vi "main.vi"() -> ()   [LabVIEW 2015]
panel:
  out "Lines Cleared":dbl
  out "score":dbl
  out "rotation":dbl
  in  "Stop":bool
  out "Stop Variable":bool
  out "X Direction":i32
  out "Y Direction":i32
  out "Array":bool[][](array[boolean])
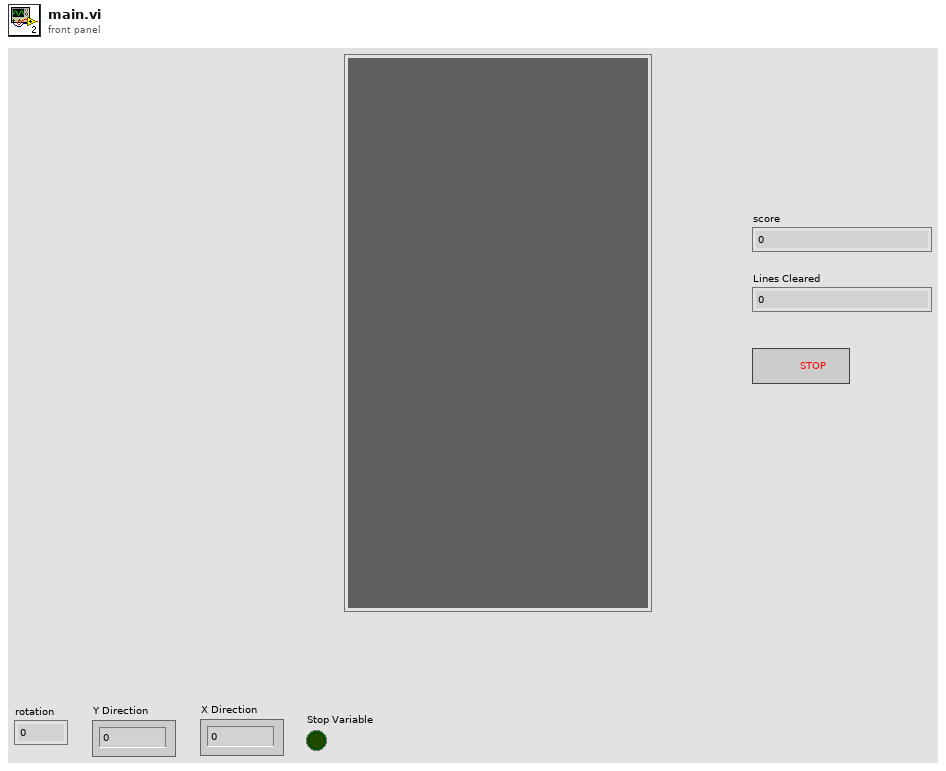
[diagram p1: front panel]
types:
  T1 = typedef "eventvkey.ctl" = enum16{"ASCII", "Enter", "Return", "Shift", "Ctrl", "Alt", "Cmd", "Opt", "Caps", "NumLock", "Clear", "Break", "Up", "Down", "Left", "Right", "Insert", "Delete", "Home", "End", "PageUp", "PageDown", "Escape", "Help", "Pause", "ScrollLock", "F1", "F2", "F3", "F4", "F5", "F6", "F7", "F8", "F9", "F10", "F11", "F12", "F13", "F14", "F15", "F16", "F17", "F18", "F19", "F20", "F21", "F22", "F23", "F24", "Play", "VolumeUp", "VolumeDown", "Mute", "Two Byte Char"}
  T2 = typedef "block.ctl" = cluster{"points":dbl[][], "type":u16, "orientaion":u16}
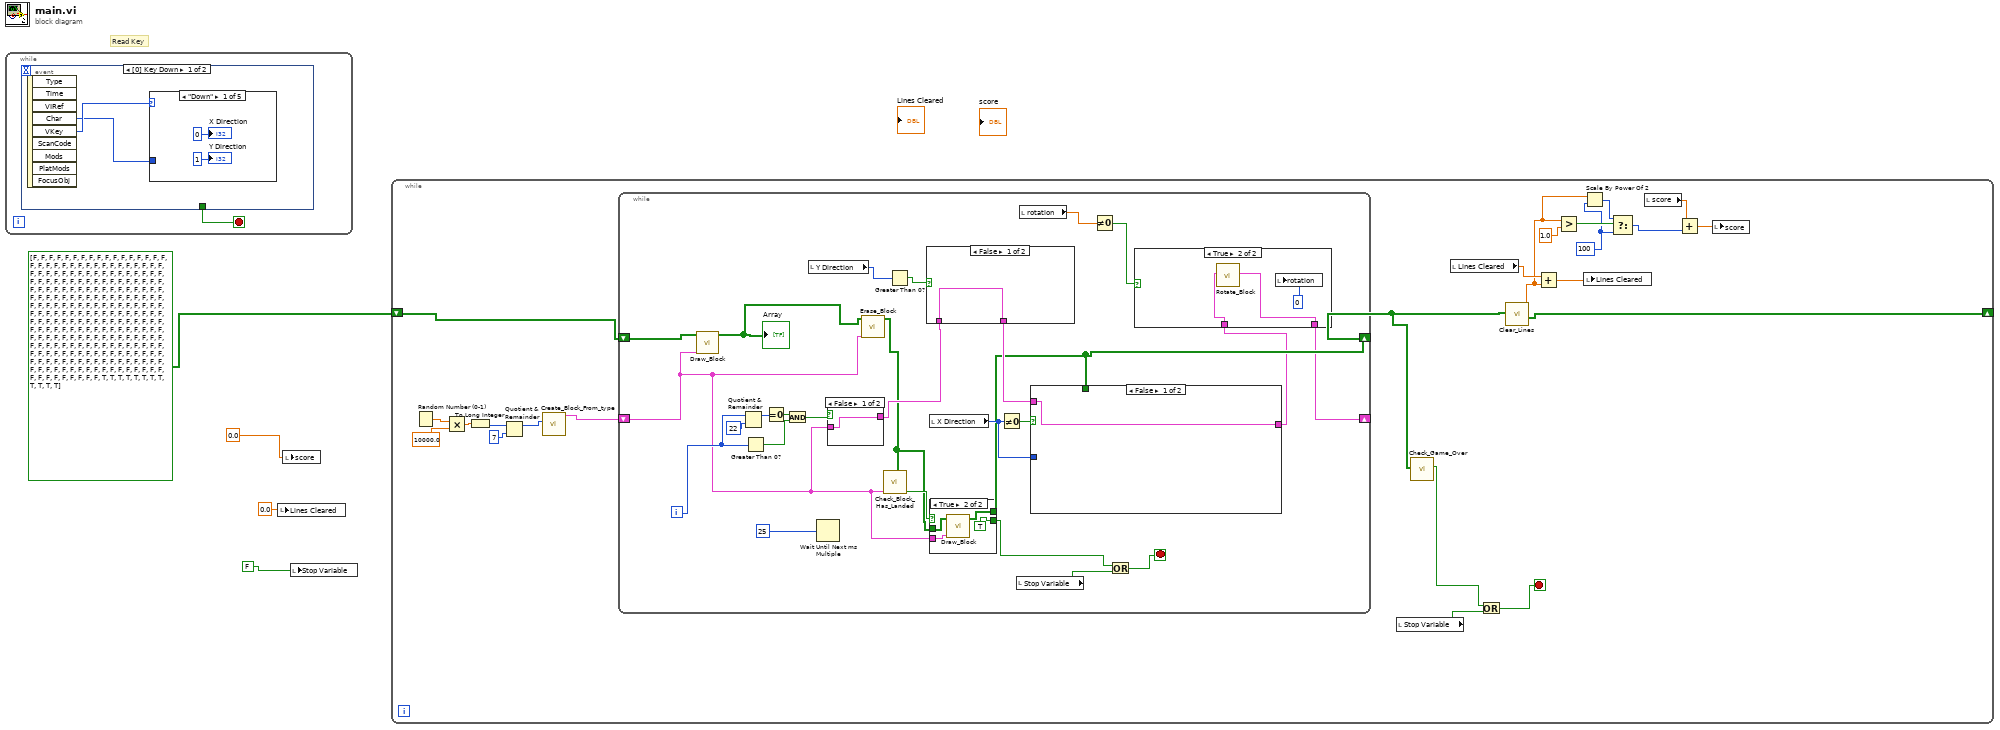
[diagram p0: block diagram]
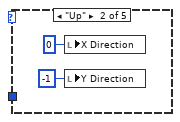
[diagram p2: hidden frame]
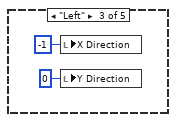
[diagram p3: hidden frame]
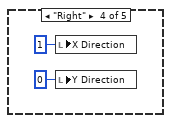
[diagram p4: hidden frame]
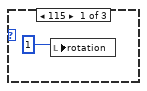
[diagram p6: hidden frame]
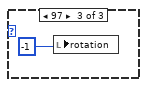
[diagram p7: hidden frame]
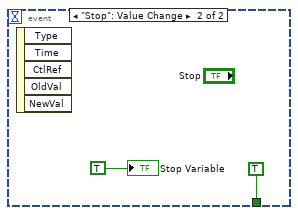
[diagram p8: hidden frame]
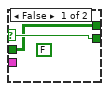
[diagram p10: hidden frame]
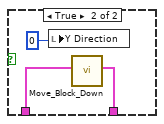
[diagram p11: hidden frame]
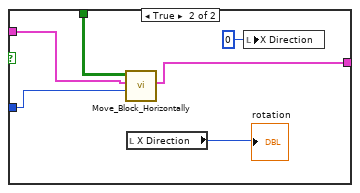
[diagram p12: hidden frame]
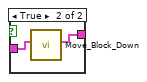
[diagram p13: hidden frame]
diagram:
  # "Read Key"
  n1 = while {
    stop <- w5 stop-if-true
    n2 = event shown="[0] Key Down" {
      selector: _ -> [_ _]
      dyn-events: _ -> [_ _]
      timeout: _ -> [_ _]
      tunnel: [_ TRUE] -> w5
      event Key Down {
        n3 = event-data() -> ("Char"=w6:i16, "VKey"=w7:T1)  [unwired: 1 in, 7 out]
        n4 = case shown="\"Down\"" w7 {
          tunnel: w6 -> [_ _ _ _ w16]
          frame "Down" {
            "X Direction" <- 0 ("X Direction")
            "Y Direction" <- 1 ("Y Direction")
          }
          frame "Up" {
            n5 = local write "X Direction"(0 ("X Direction")) -> ()
            n6 = local write "Y Direction"(-1 ("Y Direction")) -> ()
          }
          frame "Left" {
            n7 = local write "X Direction"(-1 ("X Direction")) -> ()
            n8 = local write "Y Direction"(0 ("Y Direction")) -> ()
          }
          frame "Right" {
            n9 = local write "X Direction"(1 ("X Direction")) -> ()
            n10 = local write "Y Direction"(0 ("Y Direction")) -> ()
          }
          frame "End", Default {
            n11 = case shown="0, Default" w16 {
              frame 115 {
                n12 = local write "rotation"(1 ("Y Direction")) -> ()
              }
              frame 0, Default {
              }
              frame 97 {
                n13 = local write "rotation"(-1 ("Y Direction")) -> ()
              }
            }
          }
        }
      }
      event "Stop": Value Change {
        n14 = event-data() -> ()  [unwired: 1 in, 5 out]
        "Stop Variable" <- TRUE
      }
    }
  }
  n15 = local write "Lines Cleared"(0.0) -> ()
  n16 = local write "score"(0.0) -> ()
  n17 = local write "Stop Variable"(FALSE) -> ()
  n18 = while {
    shift-right: [w35] -> _
    shift-left: bool[][] [[FALSE, FALSE, FALSE, FALSE, FALSE, FALSE, FALSE, FALSE, FALSE, FALSE, FALSE, FALSE], [FALSE, FALSE, FALSE, FALSE, FALSE, FALSE, FALSE, FALSE, FALSE, FALSE, FALSE, FALSE], [FALSE, FALSE, FALSE, FALSE, FALSE, FALSE, FALSE, FALSE, FALSE, FALSE, FALSE, FALSE], [FALSE, FALSE, FALSE, FALSE, FALSE, FALSE, FALSE, FALSE, FALSE, FALSE, FALSE, FALSE], [FALSE, FALSE, FALSE, FALSE, FALSE, FALSE, FALSE, FALSE, FALSE, FALSE, FALSE, FALSE], [FALSE, FALSE, FALSE, FALSE, FALSE, FALSE, FALSE, FALSE, FALSE, FALSE, FALSE, FALSE], [FALSE, FALSE, FALSE, FALSE, FALSE, FALSE, FALSE, FALSE, FALSE, FALSE, FALSE, FALSE], [FALSE, FALSE, FALSE, FALSE, FALSE, FALSE, FALSE, FALSE, FALSE, FALSE, FALSE, FALSE], [FALSE, FALSE, FALSE, FALSE, FALSE, FALSE, FALSE, FALSE, FALSE, FALSE, FALSE, FALSE], [FALSE, FALSE, FALSE, FALSE, FALSE, FALSE, FALSE, FALSE, FALSE, FALSE, FALSE, FALSE], [FALSE, FALSE, FALSE, FALSE, FALSE, FALSE, FALSE, FALSE, FALSE, FALSE, FALSE, FALSE], [FALSE, FALSE, FALSE, FALSE, FALSE, FALSE, FALSE, FALSE, FALSE, FALSE, FALSE, FALSE], [FALSE, FALSE, FALSE, FALSE, FALSE, FALSE, FALSE, FALSE, FALSE, FALSE, FALSE, FALSE], [FALSE, FALSE, FALSE, FALSE, FALSE, FALSE, FALSE, FALSE, FALSE, FALSE, FALSE, FALSE], [FALSE, FALSE, FALSE, FALSE, FALSE, FALSE, FALSE, FALSE, FALSE, FALSE, FALSE, FALSE], [FALSE, FALSE, FALSE, FALSE, FALSE, FALSE, FALSE, FALSE, FALSE, FALSE, FALSE, FALSE], [FALSE, FALSE, FALSE, FALSE, FALSE, FALSE, FALSE, FALSE, FALSE, FALSE, FALSE, FALSE], [FALSE, FALSE, FALSE, FALSE, FALSE, FALSE, FALSE, FALSE, FALSE, FALSE, FALSE, FALSE], [FALSE, FALSE, FALSE, FALSE, FALSE, FALSE, FALSE, FALSE, FALSE, FALSE, FALSE, FALSE], [FALSE, FALSE, FALSE, FALSE, FALSE, FALSE, FALSE, FALSE, FALSE, FALSE, FALSE, FALSE], [FALSE, FALSE, FALSE, FALSE, FALSE, FALSE, FALSE, FALSE, FALSE, FALSE, FALSE, FALSE], [FALSE, FALSE, FALSE, FALSE, FALSE, FALSE, FALSE, FALSE, FALSE, FALSE, FALSE, FALSE], [TRUE, TRUE, TRUE, TRUE, TRUE, TRUE, TRUE, TRUE, TRUE, TRUE, TRUE, TRUE]] -> [w37]
    stop <- w21 stop-if-true
    w28 = 100
    n19 = Random Number (0-1)() -> (number: 0 to 1=w43:dbl)
    n20 = Multiply(x=w43, y=10000.0) -> (x*y=w41:dbl)
    n21 = To Long Integer(number=w41) -> (32bit integer=w40:i32)
    n22 = Quotient & Remainder(x=w40, y=7) -> (x-y*floor(x/y)=w34:i32)  [unwired: 1 out]
    n23 = call "Create_Block_From_type.vi"("Numeric"=w34) -> ("Cluster"=w38:T2)  [unwired: 10 in]
    n24 = while {
      shift-right: [w51] -> w36
      shift-left: w37 -> [w68]
      shift-right: [w48] -> _
      shift-left: w38 -> [w52]
      i -> [w65]
      stop <- w44 stop-if-true
      n25 = call "Draw_Block.vi"("Block"=w52, "Input Array"=w68) -> ("Output Array"=w67:bool[][])  [unwired: 9 in]
      "Array" <- w67
      n26 = Quotient & Remainder(x=w65, y=22) -> (x-y*floor(x/y)=w62:i32)  [unwired: 1 out]
      n27 = Greater Than 0?(x=w65) -> (x > 0?=w61:bool)
      n28 = Equal To 0?(x=w62) -> (x = 0?=w63:bool)
      n29 = And(x=w63, y=w61) -> (x .and. y?=w66:bool)
      n30 = local read "Y Direction"() -> (w56:i32)
      n31 = Wait Until Next ms Multiple(millisecond multiple=25) -> ()  [unwired: 1 out]
      n32 = case shown="False" w66 {
        tunnel: w52 -> [w91 w93]
        tunnel: [w91 w92] -> w58
        frame False {
        }
        frame True {
          n33 = call "Move_Block_Down.vi"("old Block"=w93) -> ("new Block"=w92:T2)  [unwired: 10 in]
        }
      }
      n34 = call "Erase_Block.vi"("Block"=w52, "Input Array"=w67) -> ("Output Array"=w53:bool[][])  [unwired: 9 in]
      n35 = call "Check_Block_Has_Landed.vi"("Block"=w52, "Input Array"=w53) -> ("landed"=w54:bool)  [unwired: 9 in]
      n36 = Greater Than 0?(x=w56) -> (x > 0?=w57:bool)
      n37 = case shown="False" w57 {
        tunnel: w58 -> [w80 w82]
        tunnel: [w80 w81] -> w55
        frame False {
        }
        frame True {
          n38 = local write "Y Direction"(0) -> ()
          n39 = call "Move_Block_Down.vi"("old Block"=w82) -> ("new Block"=w81:T2)  [unwired: 10 in]
        }
      }
      n40 = local read "X Direction"() -> (w59:i32)
      n41 = case shown="True" w54 {
        selector: w54 -> [w75 _]
        tunnel: [w75 TRUE] -> w45
        tunnel: w53 -> [w74 w79]
        tunnel: w52 -> [_ w78]
        tunnel: [w74 w77] -> w51
        frame False {
          (unwired) FALSE
        }
        frame True {
          n42 = call "Draw_Block.vi"("Block"=w78, "Input Array"=w79) -> ("Output Array"=w77:bool[][])  [unwired: 9 in]
        }
      }
      n43 = Not Equal To 0?(x=w59) -> (x != 0?=w60:bool)
      n44 = local read "Stop Variable"() -> (w46:bool)
      n45 = local read "rotation"() -> (w50:dbl)
      n46 = case shown="False" w60 {
        tunnel: w55 -> [w84 w88]
        tunnel: [w84 w86] -> w49
        tunnel: w51 -> [_ w89]
        tunnel: w59 -> [_ w87]
        frame False {
        }
        frame True {
          n47 = call "Move_Block_Horizontally.vi"("direction"=w87, "oldBlock"=w88, "Array"=w89) -> ("newBlock"=w86:T2)  [unwired: 7 in, 1 out]
          n48 = local read "X Direction"() -> (→"rotation":i32)
          n49 = local write "X Direction"(0 ("Y Direction")) -> ()
        }
      }
      n50 = Not Equal To 0?(x=w50) -> (x != 0?=w47:bool)
      n51 = Or(x=w45, y=w46) -> (x .or. y?=w44:bool)
      n52 = case shown="True" w47 {
        tunnel: w49 -> [w70 w72]
        tunnel: [w70 w71] -> w48
        frame False {
        }
        frame True {
          n53 = call "Rotate_Block.vi"("oldBlock"=w72) -> ("newBlock"=w71:T2)  [unwired: 10 in]
          n54 = local write "rotation"(0) -> ()
        }
      }
    }
    n55 = local read "Stop Variable"() -> (w23:bool)
    n56 = call "Check_Game_Over.vi"("inputArray"=w36) -> ("gameOver"=w22:bool)  [unwired: 10 in]
    n57 = local read "Lines Cleared"() -> (w32:dbl)
    n58 = Or(x=w22, y=w23) -> (x .or. y?=w21:bool)
    n59 = call "Clear_Lines.vi"("inputArray"=w36) -> ("outputArray"=w35:bool[][], "lines"=w29:dbl)  [unwired: 9 in]
    n60 = Add(x=w32, y=w29) -> (x+y=w33:dbl)
    n61 = Greater?(x=w29, y=1.0) -> (0:w31:bool)
    n62 = Scale By Power Of 2(n=w29, x=w28) -> (x*2^n=w27:i32)
    n63 = local write "Lines Cleared"(w33) -> ()
    n64 = Select(t=w27, s=w31, f=w28) -> (s? t:f=w26:i32)
    n65 = local read "score"() -> (w25:dbl)
    n66 = Add(x=w25, y=w26) -> (x+y=w24:dbl)
    n67 = local write "score"(w24) -> ()
  }
